vi "SUB_GET_RTC_SFCS.vi"(2 "Stage":string, 3 "URL":string) -> (0 "DateTime":string, 1 "OK?":bool)   [LabVIEW 2011]
uses:
  data/MCSDLL.dll
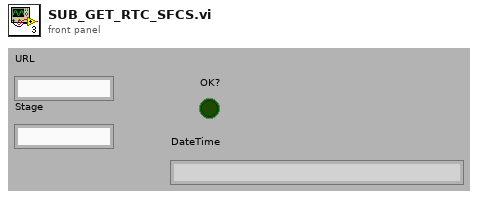
[diagram p1: front panel]
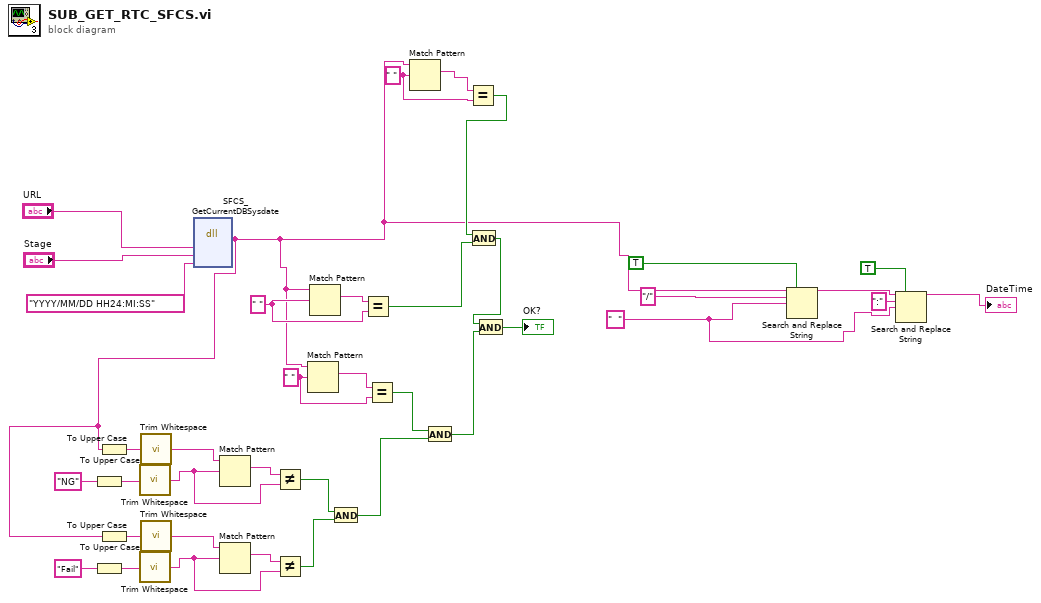
[diagram p0: block diagram]
diagram:
  w3 = "  " ("replace string (\"\")")
  w26 = " " ("regular expression")
  w28 = " " ("regular expression")
  w30 = " " ("regular expression")
  n1 = To Upper Case(1:"NG" ("string")) -> (0:w37:string)
  n2 = To Upper Case(1:"Fail" ("string")) -> (0:w19:string)
  n3 = call <vilib>:"Trim Whitespace.vi"("string"=w37) -> ("trimmed string"=w34:string)  [unwired: 1 in]
  n4 = call <vilib>:"Trim Whitespace.vi"("string"=w19) -> ("trimmed string"=w16:string)  [unwired: 1 in]
  n5 = dll-call lib="D:/S8300E_Project/data/MCSDLL.dll" fn="SFCS_GetCurrentDBSysdate"("URL"="URL", "Stage"="Stage", "TimeFormat"="YYYY/MM/DD HH24:MI:SS") -> (w8:string)  [unwired: 6 in, 2 out]
  n6 = To Upper Case(1:w8) -> (0:w38:string)
  n7 = To Upper Case(1:w8) -> (0:w20:string)
  n8 = call <vilib>:"Trim Whitespace.vi"("string"=w38) -> ("trimmed string"=w33:string)  [unwired: 1 in]
  n9 = call <vilib>:"Trim Whitespace.vi"("string"=w20) -> ("trimmed string"=w15:string)  [unwired: 1 in]
  n10 = Match Pattern(string=w33, regular expression=w34) -> (match substring=w35:string)  [unwired: 1 in, 3 out]
  n11 = Match Pattern(string=w15, regular expression=w16) -> (match substring=w17:string)  [unwired: 1 in, 3 out]
  n12 = Not Equal?(x=w35, y=w34) -> (x != y?=w14:bool)
  n13 = Not Equal?(x=w17, y=w16) -> (x != y?=w13:bool)
  n14 = Match Pattern(string=w8, regular expression=w26) -> (match substring=w27:string)  [unwired: 1 in, 3 out]
  n15 = Match Pattern(string=w8, regular expression=w28) -> (match substring=w29:string)  [unwired: 1 in, 3 out]
  n16 = And(x=w14, y=w13) -> (x .and. y?=w12:bool)
  n17 = Equal?(x=w29, y=w28) -> (x = y?=w23:bool)
  n18 = Equal?(x=w27, y=w26) -> (x = y?=w25:bool)
  n19 = Match Pattern(string=w8, regular expression=w30) -> (match substring=w31:string)  [unwired: 1 in, 3 out]
  n20 = And(x=w25, y=w12) -> (x .and. y?=w21:bool)
  n21 = Equal?(x=w31, y=w30) -> (x = y?=w24:bool)
  n22 = And(x=w24, y=w23) -> (x .and. y?=w22:bool)
  n23 = And(x=w22, y=w21) -> (x .and. y?=→"OK?":bool)
  n24 = Search and Replace String(replace all?=TRUE ("replace all? (F)"), input string=w8, search string="/", replace string=w3) -> (result string=w5:string)  [unwired: 4 in, 3 out]
  n25 = Search and Replace String(replace all?=TRUE ("replace all? (F)"), input string=w5, search string=":", replace string=w3) -> (result string=→"DateTime":string)  [unwired: 4 in, 3 out]
